vi "Disable Output.vi"(8 "error in (no error)":errorcluster, 11 "Calibrator in":refnum<class "Calibrator.lvclass">) -> (0 "error out":errorcluster, 3 "Calibrator out":refnum<class "Calibrator.lvclass">)   [LabVIEW 2015, in "Calibrator.lvclass"]
uses:
  Calibrator.lvclass
  <instrlib>/Fluke 5XXX Series Multicalibrators/Fluke 5XXX Series Multicalibrators.lvlib
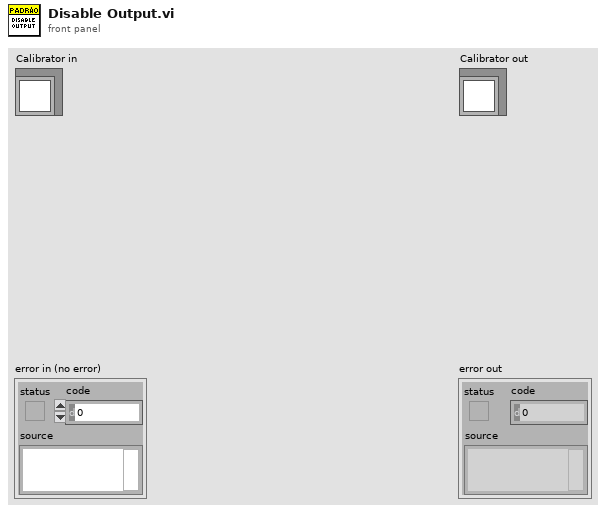
[diagram p1: front panel]
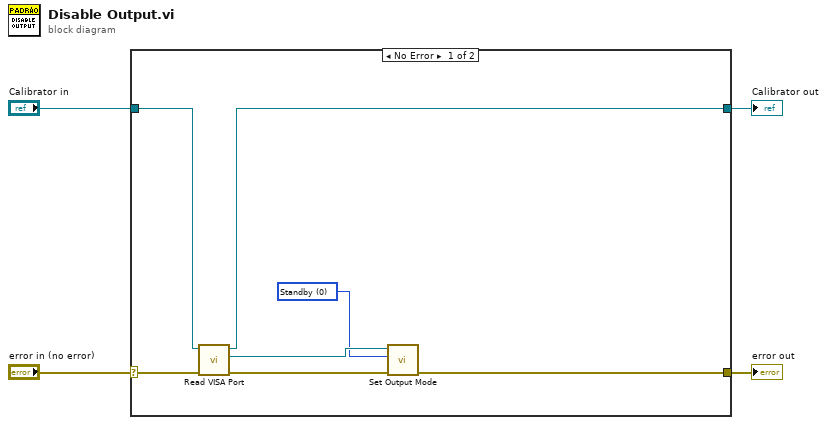
[diagram p0: block diagram]
diagram:
  n1 = case shown="No Error" "error in (no error)" {
    selector: "error in (no error)" -> [w11 w13]
    tunnel: [w5 w13] -> w3
    tunnel: [w9 w12] -> w1
    tunnel: "Calibrator in" -> [w10 w12]
    frame No Error {
      w6 = u32 0 items=["Standby", "Operate"] ("Output Mode (0: Standby)")
      n2 = call-dynamic "Read VISA Port.vi"("error in (no error)"=w11, "Device in"=w10) -> ("error out"=w7:errorcluster, "VISA Port"=w8:refnum<visa-resource-name>, "Device out"=w9:refnum<class "Calibrator.lvclass">)  [unwired: 7 in]
      n3 = call <instrlib>:"Set Output Mode.vi"("error in (no error)"=w7, "Output Mode (0: Standby)"=w6, "VISA resource name"=w8) -> ("error out"=w5:errorcluster)  [unwired: 7 in, 1 out]
    }
    frame Error {
    }
  }
  "error out" <- w3
  "Calibrator out" <- w1
